vi "_Server Start Run.vi"(2 "Error in":errorcluster, 3 "Run Method":string, 4 "Eng Refnum":refnum<vi>) -> (0 "error out":errorcluster, 1 "MethodStream#":u8)   [LabVIEW 2015]
uses:
  Configuration/AcquisitionState.ctl
  _Server Global.vi
  Configuration/_Global Configuration.vi
  LCDriver/_Global LC Driver.vi
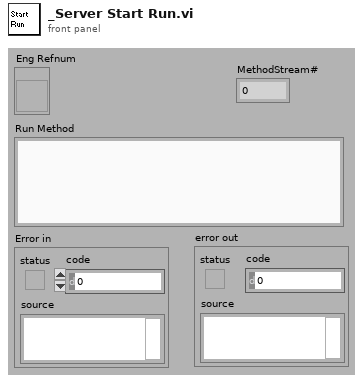
[diagram p1: front panel]
types:
  T1 = typedef "_XML Lens.ctl" = cluster{"Value":dbl, "ChID":u8}
  T2 = typedef "_Server Method.ctl" = cluster{"RunMode":i32, "Sync":u8, "Expt":T3[], "EqTime(mS)":i32, "TuneParam":T7[]}
  T3 = typedef "_XML Expt.ctl" = cluster{"StartT(mS)":i32, "#Cycles":i32, "PauseT(uS)":i32, "ScanType":i32, "Polarity":u8, "FixedMass":dbl, "DelayT(mS)":i32, "Active Ch":T1[], "Mass Range":T4[]}
  T4 = typedef "_Mass Range Property.ctl" = cluster{"Start":dbl, "Stop":dbl, "Step Size":dbl, "Steps":i32, "Dwell":dbl, "Parameters":T5[], "Res":T6}
  T5 = typedef "_Mass Range Parameters.ctl" = cluster{"Name":string, "Ch#":u8, "StartV":dbl, "StopV":dbl, "StepV":dbl, "Index":u8}
  T6 = typedef "_RT Res Type.ctl" = u16
  T7 = typedef "_RT Active Ch.ctl" = cluster{"Start":i32, "Step":i32, "ChID":i32}
  T8 = typedef "AcquisitionState.ctl" = enum16{"Ready", "Waiting", "Busy"}
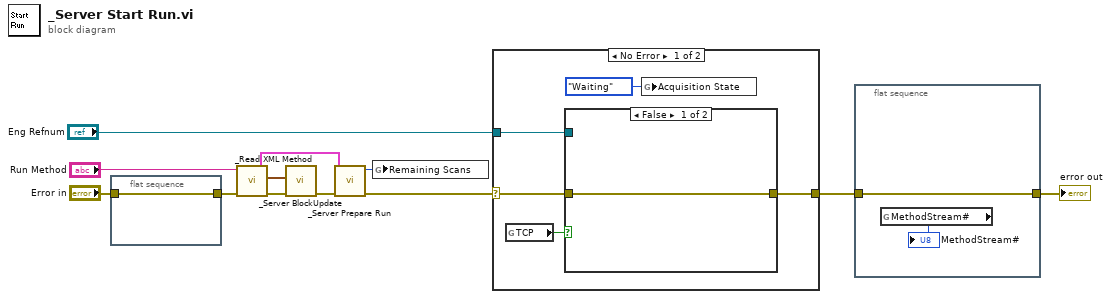
[diagram p0: block diagram]
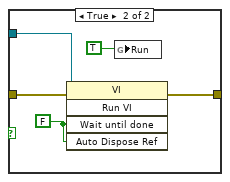
[diagram p2: hidden frame]
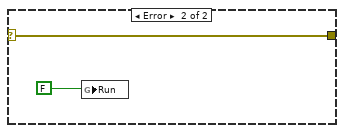
[diagram p3: hidden frame]
diagram:
  n1 = flat-sequence {
    tunnel: [w13] -> w4
    tunnel: "Error in" -> [w13]
    frame #0 {
    }
  }
  n2 = call "_Read XML Method.vi"("error in"=w4, "XML String"="Run Method") -> ("error out"=w7:errorcluster, "Lens"=w8:T1[], "Server Method"=w10:T2)  [unwired: 3 out]
  n3 = call "_Server BlockUpdate.vi"("error in"=w7, "Lens"=w8) -> ("error out"=w9:errorcluster)  [unwired: 1 in, 4 out]
  n4 = call "_Server Prepare Run.vi"("error in (no error)"=w9, "Server Method"=w10) -> ("error out"=w12:errorcluster, "Scans"=w6:i32)  [unwired: 8 out]
  n5 = global write "_Server Global.vi" "Remaining Scans"(w6) -> ()
  n6 = case shown="No Error" w12 {
    selector: w12 -> [w16 w26]
    tunnel: [w17 w26] -> w1
    tunnel: "Eng Refnum" -> [w18 _]
    frame No Error {
      n7 = global read "_Global Configuration.vi" "TCP"() -> (w15:bool)
      n8 = case shown="False" w15 {
        tunnel: w18 -> [_ w23]
        tunnel: [w19 w22] -> w17
        tunnel: w16 -> [w19 w21]
        frame False {
        }
        frame True {
          w24 = FALSE ("Wait until done")
          n9 = invoke class="VI" method="Run VI"(reference=w23, error in=w21, "Wait until done"=w24, "Auto Dispose Ref"=w24) -> (error out=w22:errorcluster)  [unwired: 1 in, 4 out]
          n10 = global write "_Global Configuration.vi" "Run"(TRUE ("Update")) -> ()
        }
      }
      n11 = global write "_Global Configuration.vi" "Acquisition State"(AcquisitionState."Waiting" ("Acquisition State")) -> ()
    }
    frame Error {
      n12 = global write "_Global Configuration.vi" "Run"(FALSE ("Update")) -> ()
    }
  }
  n13 = flat-sequence {
    tunnel: [w28] -> w2
    tunnel: w1 -> [w28]
    frame #0 {
      n14 = global read "_Global LC Driver.vi" "MethodStream#"() -> (→"MethodStream#":u8)
    }
  }
  "error out" <- w2
